vi "Datasheet Get Number.vi"(1 "String":string) -> (0 "Numeric":dbl)   [LabVIEW 2011]
uses:
  <vilib>/Utility/miscctls.llb/LVDateTimeRec.ctl
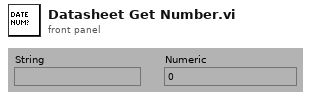
[diagram p1: front panel]
types:
  T1 = typedef "LVDateTimeRec.ctl" = cluster{"fractional second":dbl, "second":i32, "minute":i32, "hour":i32, "day of month":i32, "month":i32, "year":i32, "day of week":i32, "day of year":i32, "DST":i32}
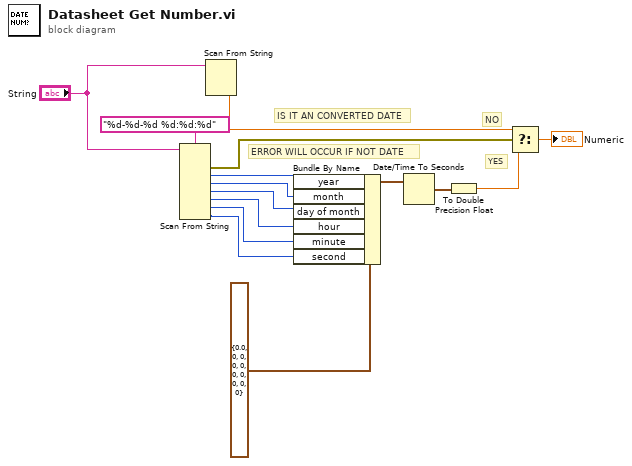
[diagram p0: block diagram]
diagram:
  # "ERROR WILL OCCUR IF NOT DATE"
  # "YES"
  # "NO"
  # "IS IT AN CONVERTED DATE"
  n1 = Scan From String(format string="%d-%d-%d %d:%d:%d", input string="String") -> (error out=w14:errorcluster, output 1=w10:i32, output 2=w9:i32, output 3=w8:i32, output 4=w7:i32, output 5=w6:i32, output 6=w5:i32)  [unwired: 2 in, 8 out]
  n2 = Scan From String(input string="String") -> (output 1=w15:dbl)  [unwired: 3 in, 4 out]
  n3 = Bundle By Name(cluster=T1 {"fractional second"=0.0, "second"=0, "minute"=0, "hour"=0, "day of month"=0, "month"=0, "year"=0, "day of week"=0, "day of year"=0, "DST"=0} ("date time rec"), "year"=w10, "month"=w9, "day of month"=w8, "hour"=w7, "minute"=w6, "second"=w5) -> (w4:T1)
  n4 = Date/Time To Seconds(2:w4) -> (0:w3:timestamp)  [unwired: 1 out]
  n5 = To Double Precision Float(number=w3) -> (double precision float=w2:dbl)
  n6 = Select(t=w15, s=w14, f=w2) -> (s? t:f=→"Numeric":dbl)
